vi "LWXPS_PositionerCorrectorSR1OffsetAccelerationGet.vi"(0 "XPS Reference IN":refnum<k24>, 7 "Positioner Name":string, 11 "LabVIEW error IN":errorcluster) -> (4 "XPS Reference OUT":refnum<k24>, 6 "Returned error code":i32, 8 "Acceleration Offset":dbl, 10 "XPS Error String":string, 15 "LabVIEW error OUT":errorcluster)   [LabVIEW 2014]
uses:
  D:/XPSQ8_LabView_Library/Development/Source/Dll/Newport.XPS.CommandInterface.dll
  Dll/Newport.XPS.CommandInterface.dll
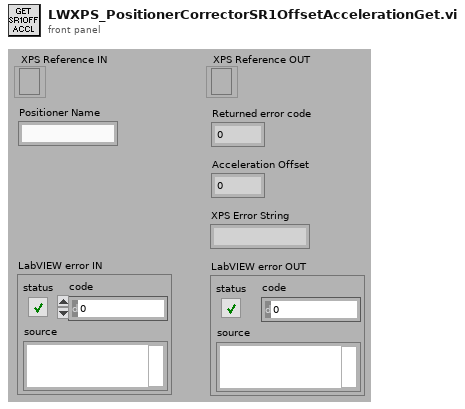
[diagram p1: front panel]
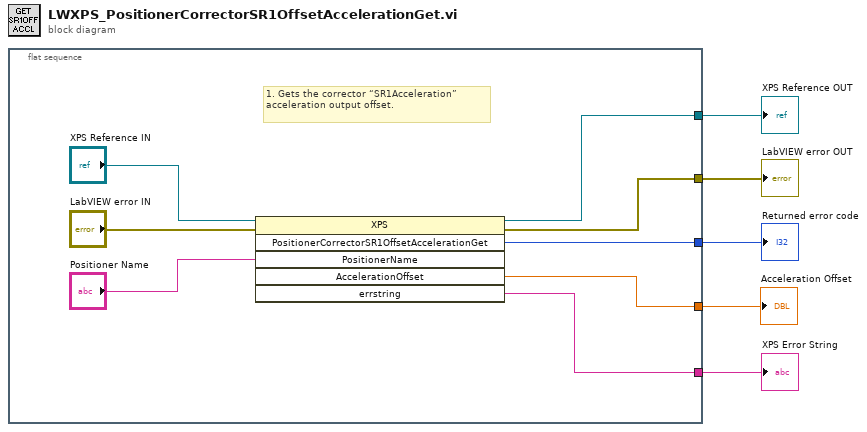
[diagram p0: block diagram]
diagram:
  n1 = flat-sequence {
    tunnel: [w11] -> w5
    tunnel: [w6] -> w4
    tunnel: [w12] -> w3
    tunnel: [w8] -> w2
    tunnel: [w7] -> w1
    frame #0 {
      # "1. Gets the corrector “SR1Acceleration” acceleration output offset."
      n2 = invoke class="XPS" method="PositionerCorrectorSR1OffsetAccelerationGet"(reference="XPS Reference IN", error in="LabVIEW error IN", "PositionerName"="Positioner Name") -> (reference out=w11:refnum<k24>, error out=w6:errorcluster, "PositionerCorrectorSR1OffsetAccelerationGet"=w12:i32, "AccelerationOffset"=w7:dbl, "errstring"=w8:string)  [unwired: 3 in, 1 out]
    }
  }
  "XPS Error String" <- w2
  "XPS Reference OUT" <- w5
  "LabVIEW error OUT" <- w4
  "Returned error code" <- w3
  "Acceleration Offset" <- w1
